vi "Encode string.vi"(7 "Field Number":i32, 10 "string":string, 11 "Buffer in":u8[](array[numeric]) format="%.0x") -> (3 "Buffer":u8[](array[numeric]) format="%.0x")   [LabVIEW 2020, in "LV-Proto.lvlib"]
uses:
  LV-Proto.lvlib
  Wire Encode Tag.vi
  Encode LEN.vi
  Wire Encode Varint I32.vi
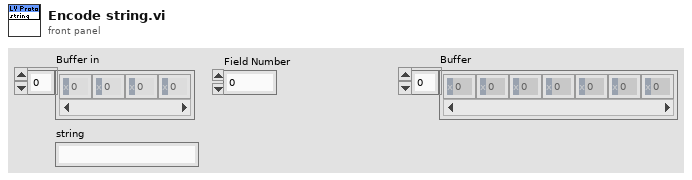
[diagram p1: front panel]
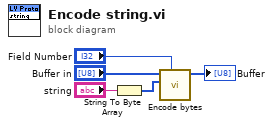
[diagram p0: block diagram]
diagram:
  n1 = String To Byte Array(string="string") -> (unsigned byte array=w3:u8[])
  n2 = call "Encode bytes.vi"("Field Number"="Field Number", "bytes"=w3, "Buffer in"="Buffer in") -> ("Buffer"=→"Buffer":u8[])  [unwired: 8 in]
